vi "ShooterMech.vi"   [LabVIEW 2015]
types:
  T1 = typedef "WPI_JoystickDevRef.ctl" = cluster{"Device":T2}
  T2 = typedef "WPI_JoystickDeviceEnum.ctl" = enum16{"USB 0", "USB 1", "USB 2", "USB 3", "USB 4", "USB 5"}
  T3 = cluster{"Buttons[0]":bool, "Buttons[1]":bool, "Buttons[2]":bool, "Buttons[3]":bool, "Buttons[4]":bool, "Buttons[5]":bool, "Buttons[6]":bool, "Buttons[7]":bool, "Buttons[8]":bool}
  T4 = typedef "WPI_MotorControlDeviceRef.ctl" = cluster{"DeviceStatus":errorcluster, "Type":T5, "PWM":cluster{"PWM Channel":T6, "DeadBand":T7}, "CAN":cluster{"Device Number":u8, "Control Mode":T8, "Semaphore":T9, "Max Vout":dbl, "TalonSRX Control Mode":T10}, "Invert":bool}
  T5 = typedef "WPI_MotorControlType.ctl" = enum16{"PWM", "CAN", "CANTalonSRX"}
  T6 = typedef "FPGA_DIOPWMChannel.ctl" = enum8{"PWM 0", "PWM 1", "PWM 2", "PWM 3", "PWM 4", "PWM 5", "PWM 6", "PWM 7", "PWM 8", "PWM 9", "PWM MXP 0", "PWM MXP 1", "PWM MXP 2", "PWM MXP 3", "PWM MXP 4", "PWM MXP 5", "PWM MXP 6", "PWM MXP 7", "PWM MXP 8", "PWM MXP 9", "Invalid"}
  T7 = typedef "WPI_PWMDeadband.ctl" = cluster{"Name":string, "maxPositivePwm":i32, "minPositivePwm":i32, "centerPwm":i32, "maxNegativePwm":i32, "minNegativePwm":i32, "angularRange":u16}
  T8 = typedef "WPI_CANJaguar_ControlMode.ctl" = enum8{"Percent VBus", "Current", "Speed", "Position", "Voltage"}
  T9 = typedef "Semaphore RefNum" = refnum<k1>
  T10 = typedef "WPI_CANTalonSRX_APIControlMode.ctl" = enum8{"Percent VBus", "Speed", "Position", "Slave", "Unchanged / Invalid", "Voltage Compensation", "Current", "Motion Profile"}
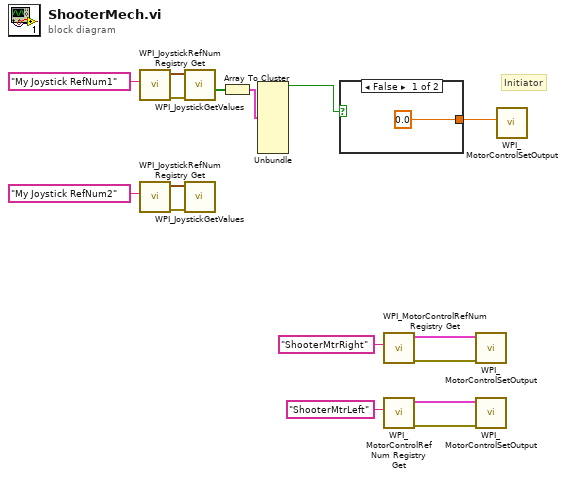
[diagram p0: block diagram]
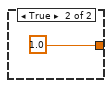
[diagram p2: hidden frame]
diagram:
  # "Initiator"
  n1 = call <vilib>:"WPI_JoystickRefNum Registry Get.vi"("refnum name"="My Joystick RefNum1") -> ("error out"=w8:errorcluster, "JoystickDevRef"=w7:T1)  [unwired: 9 in]
  n2 = call <vilib>:"WPI_JoystickRefNum Registry Get.vi"("refnum name"="My Joystick RefNum2") -> ("error out"=w6:errorcluster, "JoystickDevRef"=w5:T1)  [unwired: 9 in]
  n3 = call <vilib>:"WPI_JoystickGetValues.vi"("error in (no error)"=w8, "JoystickDevRef"=w7) -> ("Buttons"=w4:bool[])  [unwired: 5 in, 4 out]
  n4 = call <vilib>:"WPI_JoystickGetValues.vi"("error in (no error)"=w6, "JoystickDevRef"=w5) -> ()  [unwired: 5 in, 5 out]
  n5 = Array To Cluster(array=w4) -> (cluster=w3:T3)
  n6 = Unbundle(w3) -> ("Buttons[0]"=w2:bool)  [unwired: 8 out]
  n7 = case shown="False" w2 {
    tunnel: [0.0 ("Output") 1.0 ("Output")] -> w1
    frame False {
    }
    frame True {
    }
  }
  n8 = call <vilib>:"WPI_MotorControlRefNum Registry Get.vi"("refnum name"="ShooterMtrRight") -> ("error out"=w14:errorcluster, "MotorControlDevRef"=w13:T4)  [unwired: 9 in]
  n9 = call <vilib>:"WPI_MotorControlRefNum Registry Get.vi"("refnum name"="ShooterMtrLeft") -> ("error out"=w12:errorcluster, "MotorControlDevRef"=w11:T4)  [unwired: 9 in]
  n10 = call <vilib>:"WPI_MotorControlSetOutput.vi"("error in (no error)"=w14, "MotorControlDevRef"=w13) -> ()  [unwired: 7 in, 3 out]
  n11 = call <vilib>:"WPI_MotorControlSetOutput.vi"("error in (no error)"=w12, "MotorControlDevRef"=w11) -> ()  [unwired: 7 in, 3 out]
  n12 = call <vilib>:"WPI_MotorControlSetOutput.vi"("Output"=w1) -> ()  [unwired: 8 in, 3 out]
